vi "mv2v.vi"(5 "y":i32=4 min=4, 7 "WaveformIn":waveform(i16)) -> (3 "Waveform":waveform(dbl))   [LabVIEW 2010]
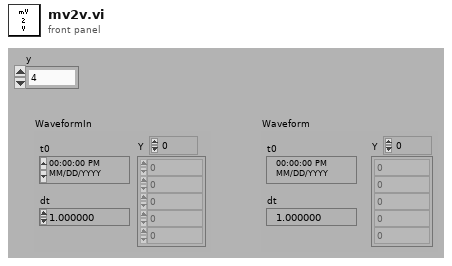
[diagram p1: front panel]
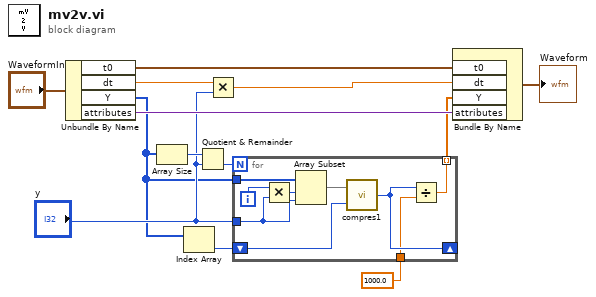
[diagram p0: block diagram]
diagram:
  n1 = Unbundle By Name("WaveformIn") -> ("t0"=w12:timestamp, "dt"=w4:dbl, "Y"=w5:i16[], "attributes"=w11:variant)
  n2 = Array Size(array=w5) -> (size(s)=w9:i32)
  n3 = Index Array(array=w5) -> (element=w7:i16)  [unwired: 1 in]
  n4 = Quotient & Remainder(x=w9, y="y") -> (floor(x/y)=w8:i32)  [unwired: 1 out]
  n5 = Multiply(x=w4, y="y") -> (x*y=w3:dbl)
  n6 = for {
    N: w8 -> [_]
    tunnel: w5 -> [w22]
    tunnel: "y" -> [w19]
    shift-right: [w16] -> _
    shift-left: w7 -> [w17]
    tunnel: [w15] -> w2 mode=indexing
    tunnel: 1000.0 -> [w14]
    i -> [w18]
    n7 = Multiply(x=w18, y=w19) -> (x*y=w20:i32)
    n8 = Array Subset(array=w22, index=w20, length=w19) -> (w21:i16[])
    n9 = call "compres1.vi"("Numeric"=w17, "Array"=w21) -> ("Numeric 2"=w16:i16)
    n10 = Divide(x=w16, y=w14) -> (x/y=w15:dbl)
  }
  n11 = Bundle By Name("t0"=w12, "dt"=w3, "Y"=w2, "attributes"=w11) -> (→"Waveform":waveform(dbl))  [unwired: 1 in]
